vi "LabVIEW Measurement UI - Post UI Update.vi"(8 "error in":errorcluster, 11 "Measurement Client Wrapper in":refnum<class "Measurement Client Wrapper.lvclass">) -> (0 "error out":errorcluster, 3 "Measurement Client Wrapper":refnum<class "Measurement Client Wrapper.lvclass">)   [LabVIEW 2020, in "Measurement Client Wrapper.lvclass"]
uses:
  Measurement Client Wrapper.lvclass
  Measurement Client Wrapper.lvclass/Measurement Client Wrapper.ctl
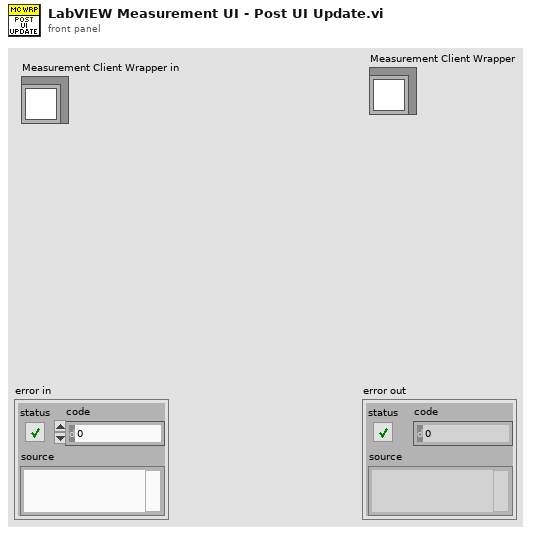
[diagram p1: front panel]
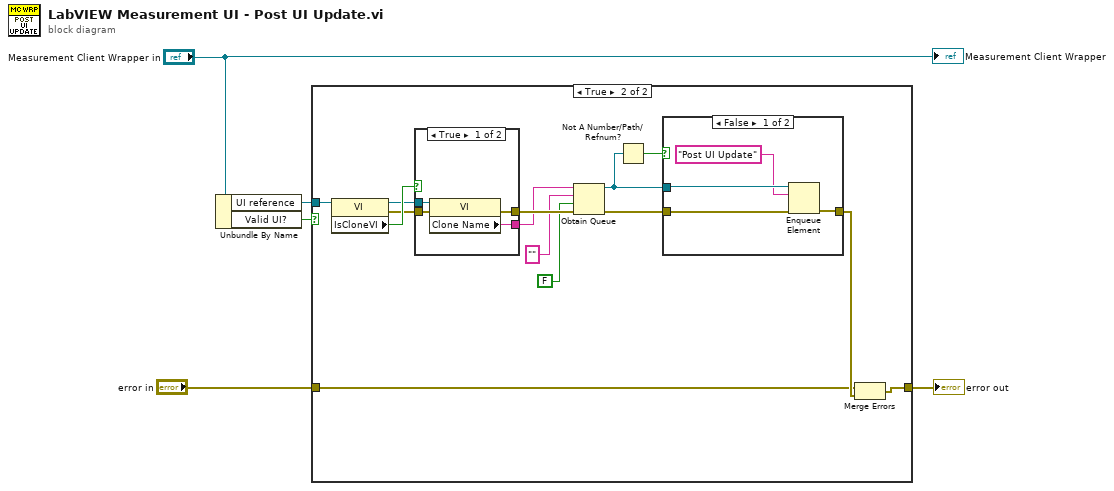
[diagram p0: block diagram]
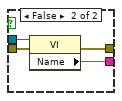
[diagram p4: hidden frame]
diagram:
  n1 = Unbundle By Name("Measurement Client Wrapper in") -> ("UI reference"=w5:refnum<vi>, "Valid UI?"=w1:bool)
  n2 = case shown="True" w1 {
    tunnel: w5 -> [_ w9]
    tunnel: [w6 w8] -> w3
    tunnel: "error in" -> [w6 w7]
    frame False {
    }
    frame True {
      n3 = property class="VI"(reference=w9) -> (reference out=w18:refnum<vi>, error out=w19:errorcluster, "IsCloneVI"=w20:bool)  [unwired: 1 in]
      n4 = case shown="True" w20 {
        tunnel: w19 -> [w29 w33]
        tunnel: w18 -> [w28 w32]
        tunnel: [w27 w31] -> w16
        tunnel: [w26 w30] -> w17
        frame True {
          n5 = property class="VI"(reference=w28, error in=w29) -> (error out=w26:errorcluster, "Clone Name"=w27:string)  [unwired: 1 out]
        }
        frame False {
          n6 = property class="VI"(reference=w32, error in=w33) -> (error out=w30:errorcluster, "Name"=w31:string)  [unwired: 1 out]
        }
      }
      n7 = Obtain Queue(name (unnamed)=w16, element data type="", create if not found? (T)=FALSE, error in (no error)=w17) -> (queue out=w11:refnum<queue>, error out=w12:errorcluster)  [unwired: 1 in, 1 out]
      n8 = Not A Number/Path/Refnum?(number/path/refnum=w11) -> (NaN/Path/Refnum?=w13:bool)
      n9 = case shown="False" w13 {
        tunnel: w12 -> [w23 w25]
        tunnel: w11 -> [w24 _]
        tunnel: [w22 w25] -> w10
        frame False {
          n10 = Enqueue Element(queue=w24, element="Post UI Update", error in (no error)=w23) -> (error out=w22:errorcluster)  [unwired: 1 in, 2 out]
        }
        frame True {
        }
      }
      n11 = Merge Errors(w7, w10) -> (w8:errorcluster)
    }
  }
  "error out" <- w3
  "Measurement Client Wrapper" <- "Measurement Client Wrapper in"
